vi "Update Method Name and Owning Folder.vi"(8 "error in":errorcluster, 9 "rpc method name":string, 10 "rpc method folder":refnum<vi>, 11 "original vi name":string) -> (0 "error out":errorcluster, 2 "owning folder":refnum<vi>, 3 "new vi name":string)   [LabVIEW 2019, in "gRPC Template Creation Utility.lvlib"]
uses:
  gRPC Template Creation Utility.lvlib
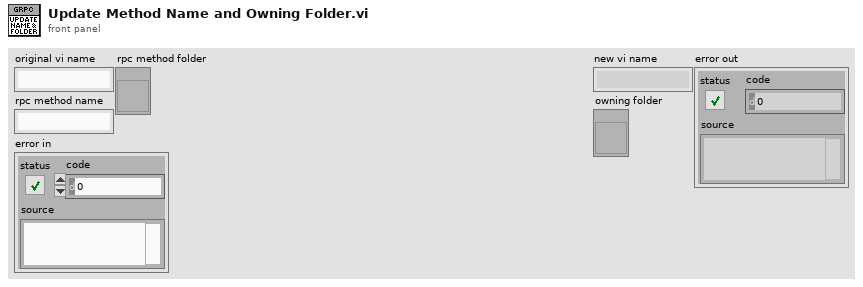
[diagram p1: front panel]
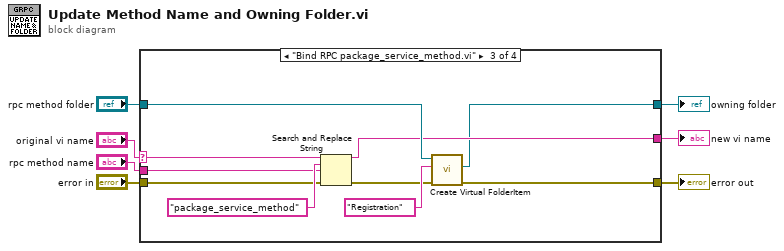
[diagram p0: block diagram]
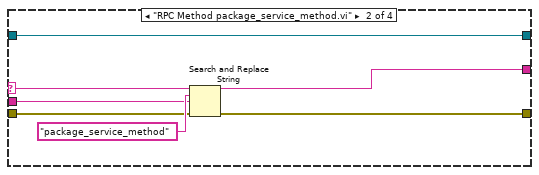
[diagram p3: hidden frame]
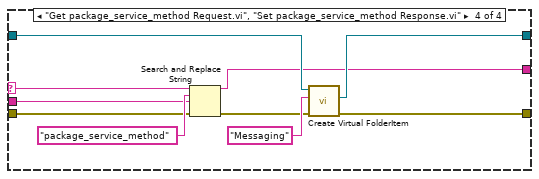
[diagram p4: hidden frame]
diagram:
  n1 = case shown="\"Bind RPC package_service_method.vi\"" "original vi name" {
    selector: "original vi name" -> [w8 w16 w26 w36]
    tunnel: "rpc method name" -> [_ w15 w25 w35]
    tunnel: "rpc method folder" -> [w9 w13 w24 w34]
    tunnel: "error in" -> [w10 w12 w21 w32]
    tunnel: [w10 w11 w18 w28] -> w1
    tunnel: [w9 w13 w19 w30] -> w2
    tunnel: [w8 w14 w22 w29] -> w3
    frame Default {
    }
    frame "RPC Method package_service_method.vi" {
      n2 = Search and Replace String(input string=w16, search string="package_service_method", replace string=w15, error in=w12) -> (result string=w14:string, error out=w11:errorcluster)  [unwired: 4 in, 2 out]
    }
    frame "Bind RPC package_service_method.vi" {
      n3 = Search and Replace String(input string=w26, search string="package_service_method", replace string=w25, error in=w21) -> (result string=w22:string, error out=w20:errorcluster)  [unwired: 4 in, 2 out]
      n4 = call "Create Virtual FolderItem.vi"("error in (no error)"=w20, "Folder Name"="Registration" ("name or relative path"), "ProjectItem in"=w24) -> ("error out"=w18:errorcluster, "FolderItem reference out"=w19:refnum<vi>)  [unwired: 5 in, 2 out]
    }
    frame "Get package_service_method Request.vi", "Set package_service_method Response.vi" {
      n5 = Search and Replace String(input string=w36, search string="package_service_method", replace string=w35, error in=w32) -> (result string=w29:string, error out=w31:errorcluster)  [unwired: 4 in, 2 out]
      n6 = call "Create Virtual FolderItem.vi"("error in (no error)"=w31, "Folder Name"="Messaging" ("name or relative path"), "ProjectItem in"=w34) -> ("error out"=w28:errorcluster, "FolderItem reference out"=w30:refnum<vi>)  [unwired: 5 in, 2 out]
    }
  }
  "new vi name" <- w3
  "owning folder" <- w2
  "error out" <- w1
